vi "Write Application.vi"(10 "Application":T1={"Loop Period (ms)"=100} {"Loop Period (ms)" min=1 max=5000}, 11 "Application in":refnum<class "Application.lvclass">) -> (3 "Application out":refnum<class "Application.lvclass">)   [LabVIEW 2013, in "Application.lvlib" / "Application.lvclass"]
uses:
  <userlib>/Common/Component/Application/Application/Application.lvclass
  <userlib>/Common/Component/Application/Configuration/Application.ctl
  <userlib>/Common/Component/Application/Application/Application.lvclass/Application.ctl
  <userlib>/Common/Component/Application/Application.lvlib
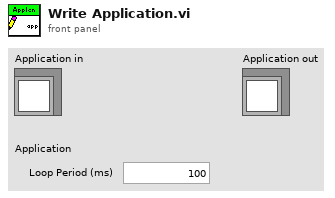
[diagram p1: front panel]
types:
  T1 = typedef "Application.lvlib/Application.ctl" = cluster{"Loop Period (ms)":u16}
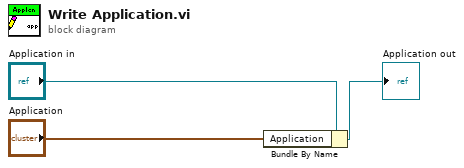
[diagram p0: block diagram]
diagram:
  n1 = Bundle By Name(cluster="Application in", "Application"="Application") -> (→"Application out":refnum<class "Application.lvclass">)
